vi "getMethods.vi"(0 "reference":refnum<class "ClassNode.lvclass">, 5 "error in (no error)":errorcluster) -> (14 "reference out":refnum<class "ClassNode.lvclass">, 15 "methods":refnum<class "MultiLineString.lvclass">, 19 "error out":errorcluster)   [LabVIEW 2014, in "ClassNode.lvclass"]
doc: "public MultiLineString getMethods()"
uses:
  <resource>/Framework/Providers/Open_GDS/UML/ClassNode_class/ClassNode.lvclass
  <resource>/Framework/Providers/Open_GDS/UML/MultiLineString_class/MultiLineString.lvclass
panel:
  # "Always set\nVI Server class\nto current VI. Do not\nconnect this control\nto the connector pane.\n(Tip!: Just drag\nand drop the icon\ninto the refnum)"
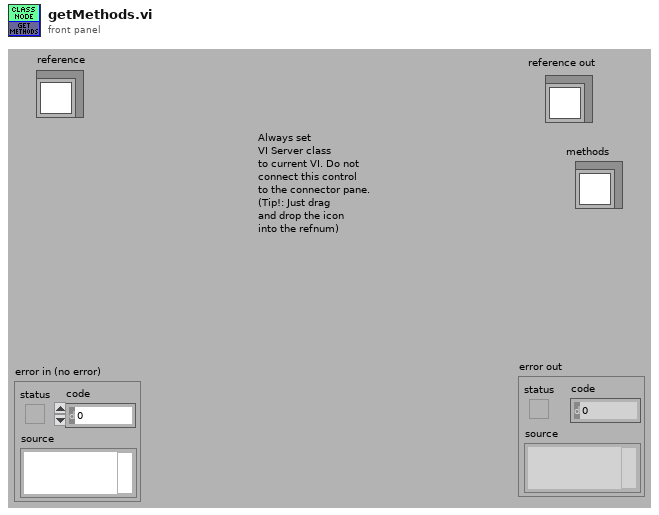
[diagram p1: front panel]
types:
  T1 = typedef "ClassNode.lvclass/ObjectAttributes.ctl" = cluster{"Base class":T2, "midHeight":dbl, "botHeight":dbl, "name":refnum<class "MultiLineString.lvclass">, "attributes":refnum<class "MultiLineString.lvclass">, "methods":refnum<class "MultiLineString.lvclass">, "DEFAULT_COMPARTMENT_HEIGHT":i32, "DEFAULT_WIDTH":i32, "DEFAULT_HEIGHT":i32, "showMethods":bool, "showAttributes":bool, "ClassPath":path}
  T2 = typedef "RectangularNode.lvclass/ObjectAttributes.ctl" = cluster{"Base class":T3, "bounds":T4}
  T3 = typedef "AbstractNode.lvclass/ObjectAttributes.ctl" = cluster{"parent":refnum<class "AbstractNode.lvclass">, "children":refnum<class "AbstractNode.lvclass">[], "Hidden":bool}
  T4 = typedef "Rectangle Rectangle2D.ctl" = cluster{"x":dbl, "y":dbl, "width":dbl, "height":dbl}
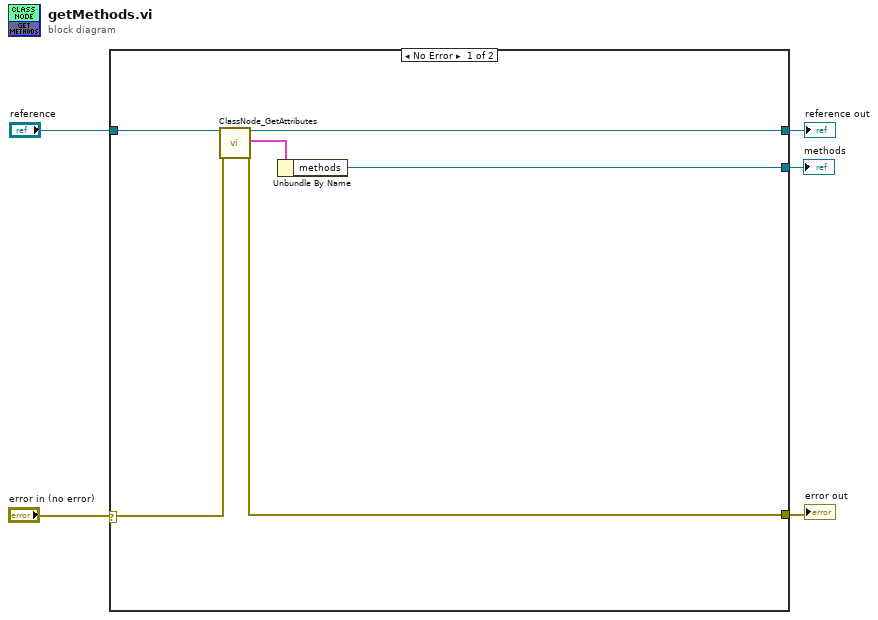
[diagram p0: block diagram]
diagram:
  n1 = case shown="No Error" "error in (no error)" {
    selector: "error in (no error)" -> [w6 w12]
    tunnel: "reference" -> [w11 w13]
    tunnel: [w10 w12] -> w4
    tunnel: [w9 w13] -> w3
    tunnel: [w8 _] -> w1
    frame No Error {
      n2 = call <resource>:"ClassNode_GetAttributes.vi"("reference in"=w11, "error in (no error)"=w6) -> ("reference out"=w9:refnum<class "ClassNode.lvclass">, "Attributes"=w7:T1, "error out"=w10:errorcluster)  [unwired: 15 out]
      n3 = Unbundle By Name(w7) -> ("methods"=w8:refnum<class "MultiLineString.lvclass">)
    }
    frame Error {
    }
  }
  "reference out" <- w3
  "error out" <- w4
  "methods" <- w1
